vi "MGI Time Format String Handle Period.vi"(11 "String[]":string[](array[string])=["1.32.23", "45 ", "12:23:34.34", "Wednesday, April 4"]) -> (3 "Separated String[]":string[](array[string]))   [LabVIEW 2016]
doc: "This VI is used by MGI Determine Time Format String to handle using a <B>.</B> as a date separator. Normally, the <B>.</B> is used for time: 12:03:34.34 pm.\nHowever, it may be used with a date: 12.31.2010\nThis VI will further separate the separated strings if the <B>.</B> is used without a preceding <B>:</B>.\n\nAuthored by Shawn Walpole\nsupport@mooregoodideas.com\nwww.mooregoodideas.com\n\nCopyright (c) 2010, Moore Good Ideas, Inc.\n\nAll rights reserved.\n\nRedistribution and use in source and binary forms, with or without modification, are permitted provided that the following conditions are met:\n\n * Redistributions of source code must retain the above copyright notice, this list of conditions and the following disclaimer.\n * Redistributions in binary form must reproduce the above copyright notice, this list of conditions and the following disclaimer in the documentation and/or other materials provided with the distribution.\n * Neither the name of Moore Good Ideas, Inc. nor the names of its contributors may be used to endorse or promote products derived from this software without specific prior written permission.\n\nTHIS SOFTWARE IS PROVIDED BY THE COPYRIGHT HOLDERS AND CONTRIBUTORS \"AS IS\" AND ANY EXPRESS OR IMPLIED WARRANTIES, INCLUDING, BUT NOT LIMITED TO, THE IMPLIED WARRANTIES OF MERCHANTABILITY AND FITNESS FOR A PARTICULAR PURPOSE ARE DISCLAIMED. IN NO EVENT SHALL THE COPYRIGHT OWNER OR CONTRIBUTORS BE LIABLE FOR ANY DIRECT, INDIRECT, INCIDENTAL, SPECIAL, EXEMPLARY, OR CONSEQUENTIAL DAMAGES (INCLUDING, BUT NOT LIMITED TO, PROCUREMENT OF SUBSTITUTE GOODS OR SERVICES; LOSS OF USE, DATA, OR PROFITS; OR BUSINESS INTERRUPTION) HOWEVER CAUSED AND ON ANY THEORY OF LIABILITY, WHETHER IN CONTRACT, STRICT LIABILITY, OR TORT (INCLUDING NEGLIGENCE OR OTHERWISE) ARISING IN ANY WAY OUT OF THE USE OF THIS SOFTWARE, EVEN IF ADVISED OF THE POSSIBILITY OF SUCH DAMAGE."
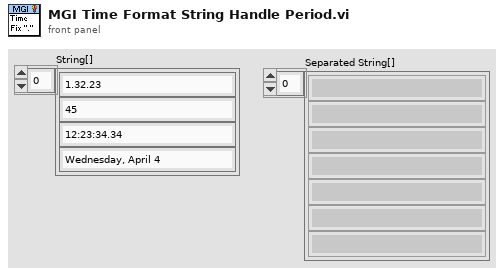
[diagram p1: front panel]
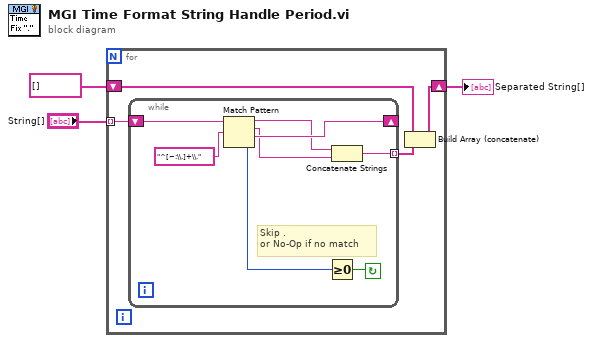
[diagram p0: block diagram]
diagram:
  n1 = for {
    tunnel: "String[]" -> [w7] mode=indexing
    shift-right: [w5] -> w1
    shift-left: string[] [] ("Separated String") -> [w6]
    n2 = while {
      shift-right: [w13] -> _
      shift-left: w7 -> [w15]
      tunnel: [w11] -> w4 mode=indexing
      stop <- w9 continue-if-true
      # "Skip .\nor No-Op if no match"
      n3 = Match Pattern(string=w15, regular expression="^[~:\\.]+\\.") -> (before substring=w12:string, match substring=w8:string, after substring=w13:string, offset past match=w10:i32)  [unwired: 1 in]
      n4 = Greater Or Equal To 0?(x=w10) -> (x >= 0?=w9:bool)
      n5 = Concatenate Strings(w12, w8) -> (w11:string)
    }
    n6 = Build Array (concatenate)(w6, w4) -> (w5:string[])
  }
  "Separated String[]" <- w1
